vi "Write Configeration Data.vi"(8 "error in":errorcluster, 9 "Volt Channel":T1={"Index"=[], "Chl Name"=[], "Scale"=[], "Offset"=[], "Sample Rate"=100, "Device Name"="", "Channel"=""}, 10 "File Refnum":variant, 11 "TDMS File in":refnum<class "TDMS File.lvclass">) -> (0 "error out":errorcluster, 3 "TDMS File out":refnum<class "TDMS File.lvclass">)   [LabVIEW 2021, in "TDMS File.lvclass"]
doc: "This vi helps to write Sample Rate, Channel Index, Channel Name, Scale and Offset into a TDMS file."
uses:
  TDMS File.lvclass
  Control/Volt Chl.ctl
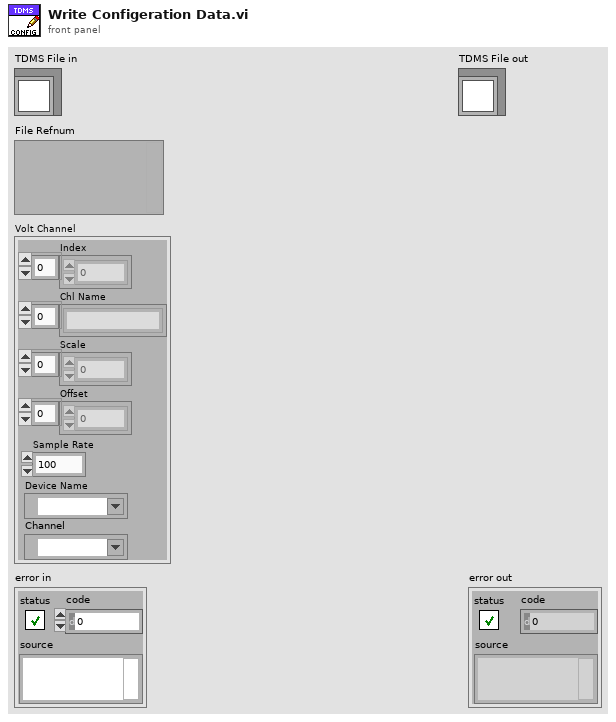
[diagram p1: front panel]
types:
  T1 = typedef "Volt Chl.ctl" = cluster{"Index":i32[], "Chl Name":string[], "Scale":dbl[], "Offset":dbl[], "Sample Rate":i32, "Device Name":tag, "Channel":tag}
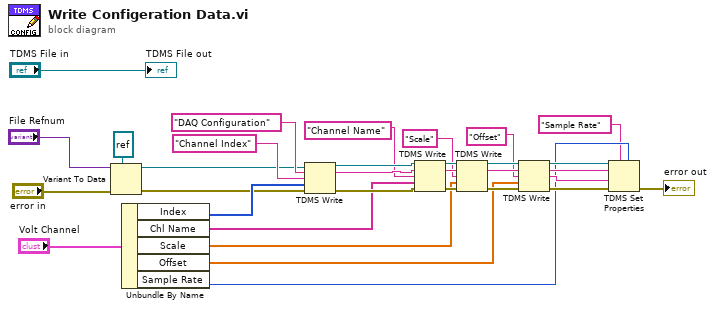
[diagram p0: block diagram]
diagram:
  n1 = Variant To Data(error in="error in", type=refnum<k34> refnum ("tdms Refnum"), Variant="File Refnum") -> (data=w6:refnum<k34>, error out=w7:errorcluster)
  n2 = Unbundle By Name("Volt Channel") -> ("Index"=w31:i32[], "Chl Name"=w4:string[], "Scale"=w20:dbl[], "Offset"=w19:dbl[], "Sample Rate"=w11:i32)
  n3 = TDMS Write(0:w6, 5:"DAQ Configuration" ("group name in (Untitled)"), 7:"Channel Index" ("group name in (Untitled)"), 9:w31, 11:w7) -> (4:w29:refnum<k34>, 6:w28:string, 15:w27:errorcluster)  [unwired: 1 in, 1 out]
  n4 = TDMS Write(0:w29, 5:w28, 7:"Channel Name" ("group name in (Untitled)"), 9:w4, 11:w27) -> (4:w25:refnum<k34>, 6:w21:string, 15:w24:errorcluster)  [unwired: 1 in, 1 out]
  n5 = TDMS Write(0:w25, 5:w21, 7:"Scale" ("group name in (Untitled)"), 9:w20, 11:w24) -> (4:w23:refnum<k34>, 6:w17:string, 15:w22:errorcluster)  [unwired: 1 in, 1 out]
  n6 = TDMS Write(0:w23, 5:w17, 7:"Offset" ("group name in (Untitled)"), 9:w19, 11:w22) -> (4:w12:refnum<k34>, 6:w13:string, 8:w14:string, 15:w15:errorcluster)  [unwired: 1 in]
  n7 = TDMS Set Properties(5:w11, 7:"Sample Rate" ("property names"), 8:w15, 9:w14, 10:w13, 11:w12) -> (0:→"error out":errorcluster)  [unwired: 3 out]
  "TDMS File out" <- "TDMS File in"
